vi "Unscramble_Multiplex_chs.vi"(1 "Channel Numbers":i16[](array[numeric]), 2 "Multiplex Ch No":i16[](array[numeric]), 3 "Voltages":dbl[][](array[numeric])) -> (0 "Voltage by Req Ch":dbl[][](array[numeric]))   [LabVIEW 2012]
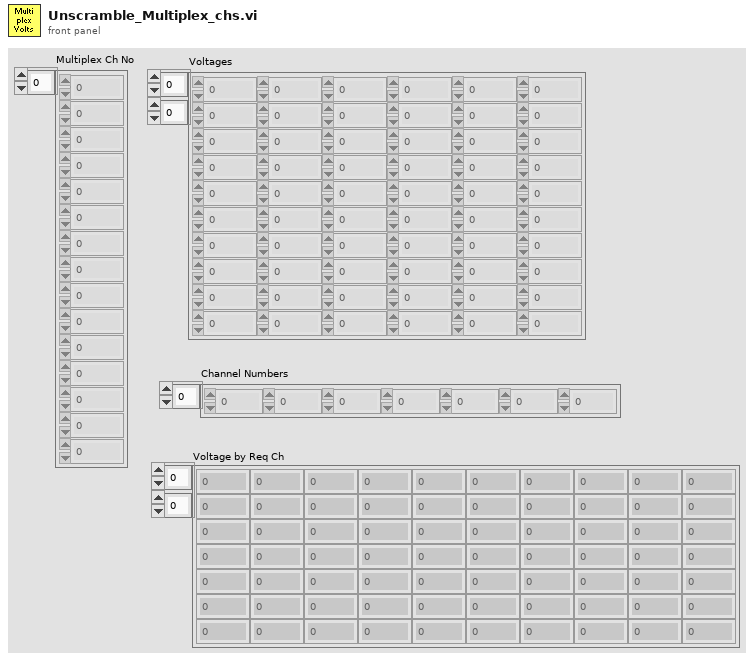
[diagram p1: front panel]
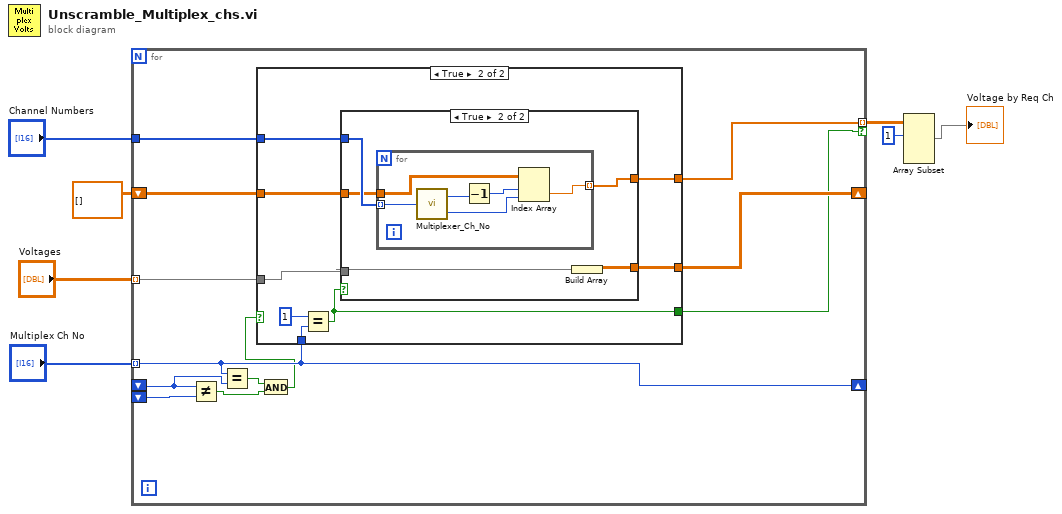
[diagram p0: block diagram]
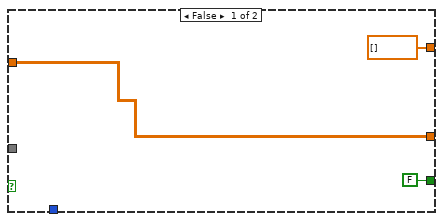
[diagram p2: hidden frame]
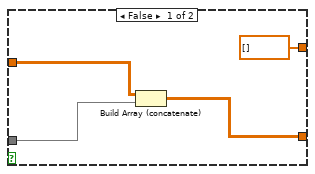
[diagram p3: hidden frame]
diagram:
  n1 = for {
    tunnel: "Multiplex Ch No" -> [w15] mode=indexing
    shift-right: [w15] -> _
    shift-left: _ -> [w18]
    shift-left: _ -> [w19]
    shift-right: [w12] -> _
    shift-left: dbl[][] [] -> [w13]
    tunnel: "Voltages" -> [w14] mode=indexing
    tunnel: "Channel Numbers" -> [w10]
    tunnel: [w9] -> w3 mode=indexing if=w8
    n2 = Not Equal?(x=w18, y=w19) -> (x != y?=w16:bool)
    n3 = Equal?(x=w15, y=w18) -> (x = y?=w17:bool)
    n4 = And(x=w17, y=w16) -> (x .and. y?=w11:bool)
    n5 = case shown="True" w11 {
      tunnel: w15 -> [_ w27]
      tunnel: w14 -> [_ w30]
      tunnel: w13 -> [w22 w29]
      tunnel: [w22 w28] -> w12
      tunnel: w10 -> [_ w25]
      tunnel: [dbl[] [] w24] -> w9
      tunnel: [FALSE w23] -> w8
      frame False {
      }
      frame True {
        n6 = Equal?(x=i16 1, y=w27) -> (x = y?=w23:bool)
        n7 = case shown="True" w23 {
          tunnel: w30 -> [w34 w39]
          tunnel: w29 -> [w33 w36]
          tunnel: [w32 w38] -> w28
          tunnel: w25 -> [_ w37]
          tunnel: [dbl[] [] w35] -> w24
          frame False {
            n8 = Build Array (concatenate)(w33, w34) -> (w32:dbl[][])
          }
          frame True {
            n9 = for {
              tunnel: w37 -> [w45] mode=indexing
              tunnel: w36 -> [w44]
              tunnel: [w42] -> w35 mode=indexing
              n10 = call "Multiplexer_Ch_No.vi"("Channel Number"=w45) -> ("Multiplexer Ch No"=w41:i16, "ADC Ch No"=w43:i16)
              n11 = Decrement(x=w41) -> (x-1=w40:i16)
              n12 = Index Array(array=w44, index (row)=w40, index (col)=w43) -> (element=w42:dbl)
            }
            n13 = Build Array(w39) -> (w38:dbl[][])
          }
        }
      }
    }
  }
  n14 = Array Subset(array=w3, index (row)=1 ("index")) -> (→"Voltage by Req Ch":dbl[][])  [unwired: 3 in]
